vi "TIFF Client Open.vi"(0 "para0":cluster{}, 1 "para4":cluster{}, 2 "para6":cluster{}, 3 "para8":cluster{}, 5 "para1":cluster{}, 7 "para2":u32, 9 "para3":cluster{}, 11 "error in (no error)":errorcluster, 12 "para5":cluster{}, 13 "para7":cluster{}, 14 "para9":cluster{}) -> (4 "function return":u32, 8 "para2 out":u32, 15 "error out":errorcluster)   [LabVIEW 2018]
doc: "LIBTIFF_DLL_IMPEXP TIFF* TIFFClientOpen(const char*, const char*,\n thandle_t,\n TIFFReadWriteProc, TIFFReadWriteProc,\n TIFFSeekProc, TIFFCloseProc,\n TIFFSizeProc,\n TIFFMapFileProc, TIFFUnmapFileProc);"
uses:
  libtiff3.dll
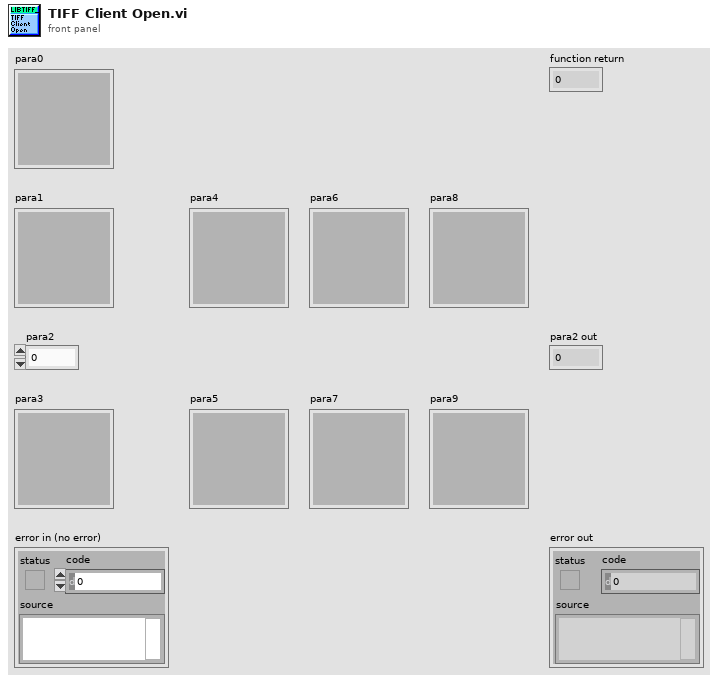
[diagram p1: front panel]
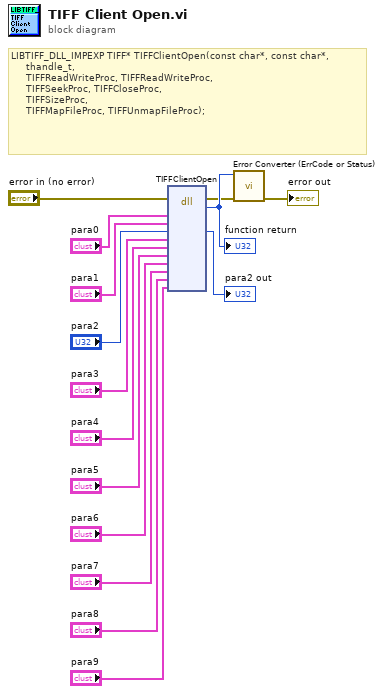
[diagram p0: block diagram]
diagram:
  # "LIBTIFF_DLL_IMPEXP\tTIFF* TIFFClientOpen(const char*, const char*,\n\t    thandle_t,\n\t    TIFFReadWriteProc, TIFFReadWriteProc,\n\t    TIFFSeekProc, TIFFCloseProc,\n\t    TIFFSizeProc,\n\t    TIFFMapFileProc, TIFFUnmapFileProc);"
  n1 = dll-call lib="C:/Users/johan/Downloads/LabVIEW software/LabVIEW software/IX-81 Software/lib/tiff/LibTiffLabview/libtiff3.*" fn="TIFFClientOpen"(error in="error in (no error)", "para0"="para0", "para1"="para1", "para2"="para2", "para3"="para3", "para4"="para4", "para5"="para5", "para6"="para6", "para7"="para7", "para8"="para8", "para9"="para9") -> (error out=w2:errorcluster, w15:u32, "para2"=→"para2 out":u32)  [unwired: 11 in, 1 out]
  "function return" <- w15
  n2 = call "Error Converter (ErrCode or Status).vi"("error in (no error)"=w2, "error code"=w15) -> ("error out"=→"error out":errorcluster)  [unwired: 9 in]
